vi "Quaternion_New_LVQuat.vi"(11 "LV quaternion":T1) -> (3 "out Quaternion":T2={"R"=1.0, "V"=[0.0, 0.0, 0.0]})   [LabVIEW 2019, in "Trajectory_Library.lvlib"]
doc: "Convenience constructors that takes in x and y values directly instead of having to construct a Translation2d.\n\nParameters:\n - X- The x component of the translational component of the pose.\n - Y - The y component of the translational component of the pose.\n - Rotation (Heading) - The rotational component of the pose.\n\nReturns:\n - OUT POSE - Output POSE"
uses:
  QUATERNION.ctl
  Trajectory_Library.lvlib
  <vilib>/robotics/Kinematics/Quaternion.ctl
  <vilib>/robotics/Kinematics/NI_Kinematics.lvlib
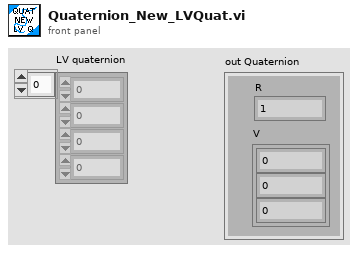
[diagram p1: front panel]
types:
  T1 = typedef "NI_Kinematics.lvlib/Quaternion.ctl" = dbl[]
  T2 = typedef "Trajectory_Library.lvlib/QUATERNION.ctl" = cluster{"R":dbl, "V":dbl[]}
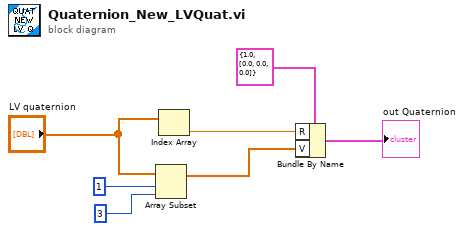
[diagram p0: block diagram]
diagram:
  n1 = Array Subset(array="LV quaternion", index=1, length=3) -> (w1:T1)
  n2 = Index Array(array="LV quaternion") -> (element=w5:dbl)  [unwired: 1 in]
  n3 = Bundle By Name(cluster=T2 {"R"=1.0, "V"=[0.0, 0.0, 0.0]} ("sumPOSE"), "R"=w5, "V"=w1) -> (→"out Quaternion":T2)
